vi "Number_Dec_Hex.vi"(0 "Dec(Any)/Hex(unsigned only) Number":string, 3 "Dec(Any)/Hex(unsigned only) Number 2":string) -> (1 "offset past number":i32, 4 "offset past number 2":i32, 5 "Numeric":dbl, 6 "Dec (True) or\nHex (False)":bool, 7 "Numeric 2":dbl, 8 "Dec (True) or\nHex (False) 2":bool)   [LabVIEW 2017]
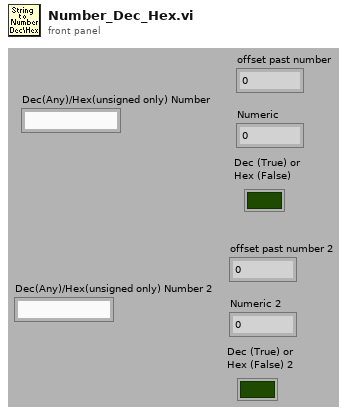
[diagram p1: front panel]
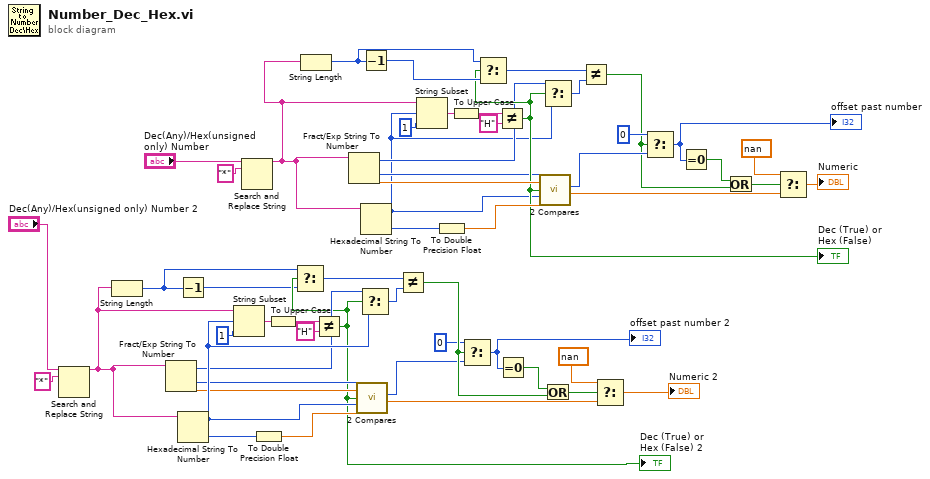
[diagram p0: block diagram]
diagram:
  n1 = Search and Replace String(input string="Dec(Any)/Hex(unsigned only) Number 2", search string="*") -> (result string=w26:string)  [unwired: 6 in, 3 out]
  n2 = String Length(string=w26) -> (length=w1:i32)
  n3 = Fract/Exp String To Number(string=w26) -> (offset past number=w20:i32, number=w7:dbl)  [unwired: 3 in]
  n4 = Decrement(x=w1) -> (x-1=w2:i32)
  n5 = Hexadecimal String To Number(string=w26) -> (offset past number=w21:i32, number=w8:u32)  [unwired: 2 in]
  n6 = String Subset(string=w26, offset (0)=w21, length (rest)=1 ("length (rest)")) -> (substring=w13:string)
  n7 = Search and Replace String(input string="Dec(Any)/Hex(unsigned only) Number", search string="*") -> (result string=w27:string)  [unwired: 6 in, 3 out]
  n8 = To Double Precision Float(number=w8) -> (double precision float=w9:dbl)
  n9 = To Upper Case(1:w13) -> (0:w11:string)
  n10 = String Length(string=w27) -> (length=w39:i32)
  n11 = Not Equal?(x=w11, y="H") -> (x != y?=w6:bool)
  "Dec (True) or\nHex (False) 2" <- w6
  n12 = Select(t=w1, s=w6, f=w2) -> (s? t:f=w18:i32)
  n13 = Fract/Exp String To Number(string=w27) -> (offset past number=w35:i32, number=w52:dbl)  [unwired: 3 in]
  n14 = call "2 Compares.vi"("InA I32"=w20, "InA DBL"=w7, "Select A/B"=w6, "InB I32"=w21, "InB DBL"=w9) -> ("Out I32"=w22:i32, "Out DBL"=w15:dbl)  [unwired: 9 in]
  n15 = Select(t=w20, s=w6, f=w21) -> (s? t:f=w19:i32)
  n16 = Decrement(x=w39) -> (x-1=w40:i32)
  n17 = Hexadecimal String To Number(string=w27) -> (offset past number=w34:i32, number=w51:u32)  [unwired: 2 in]
  n18 = Not Equal?(x=w18, y=w19) -> (x != y?=w24:bool)
  n19 = String Subset(string=w27, offset (0)=w34, length (rest)=1 ("length (rest)")) -> (substring=w46:string)
  n20 = To Double Precision Float(number=w51) -> (double precision float=w50:dbl)
  n21 = To Upper Case(1:w46) -> (0:w48:string)
  n22 = Select(t=0, s=w24, f=w22) -> (s? t:f=w4:i32)
  "offset past number 2" <- w4
  n23 = Not Equal?(x=w48, y="H") -> (x != y?=w36:bool)
  "Dec (True) or\nHex (False)" <- w36
  n24 = Select(t=w39, s=w36, f=w40) -> (s? t:f=w38:i32)
  n25 = Equal To 0?(x=w4) -> (x = 0?=w25:bool)
  n26 = call "2 Compares.vi"("InA I32"=w35, "InA DBL"=w52, "Select A/B"=w36, "InB I32"=w34, "InB DBL"=w50) -> ("Out I32"=w33:i32, "Out DBL"=w44:dbl)  [unwired: 9 in]
  n27 = Select(t=w35, s=w36, f=w34) -> (s? t:f=w37:i32)
  n28 = Or(x=w25, y=w24) -> (x .or. y?=w23:bool)
  n29 = Not Equal?(x=w38, y=w37) -> (x != y?=w30:bool)
  n30 = Select(t=nan, s=w23, f=w15) -> (s? t:f=→"Numeric 2":dbl)
  n31 = Select(t=0, s=w30, f=w33) -> (s? t:f=w32:i32)
  "offset past number" <- w32
  n32 = Equal To 0?(x=w32) -> (x = 0?=w29:bool)
  n33 = Or(x=w29, y=w30) -> (x .or. y?=w31:bool)
  n34 = Select(t=nan, s=w31, f=w44) -> (s? t:f=→"Numeric":dbl)
